vi "CheckID.vi"(8 "error in":errorcluster, 10 "CANData":T1, 11 "CAN-Frames":refnum<k21>[](array[refnum])) -> (0 "error out":errorcluster, 1 "FrameOut":T2, 2 "found？":bool)   [LabVIEW 2019, in "CAN-NI.lvlib" / "CAN-NI.lvclass"]
uses:
  CAN-NI.lvclass
  CAN-Interface/TypeDef/Def-CANData.ctl
  <resource>/objmgr/xnet.rc
  CAN-Interface/Class-Interface.lvclass
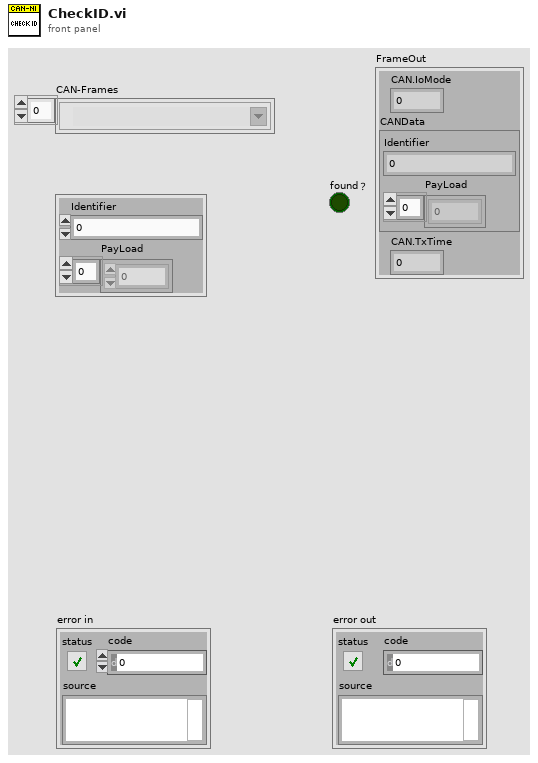
[diagram p1: front panel]
types:
  T1 = typedef "CAN-Interface.lvlib/Class-Interface.lvclass/Def-CANData.ctl" = cluster{"Identifier":u32, "PayLoad":u8[]}
  T2 = cluster{"CAN.IoMode":u32, "CANData":T1, "CAN.TxTime":dbl}
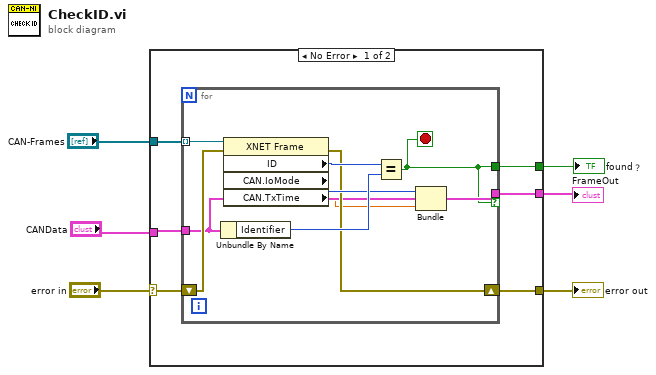
[diagram p0: block diagram]
diagram:
  n1 = case shown="No Error" "error in" {
    selector: "error in" -> [w9 w23]
    tunnel: "CAN-Frames" -> [w12 _]
    tunnel: "CANData" -> [w7 _]
    tunnel: [w11 _] -> w1
    tunnel: [w10 _] -> w5
    tunnel: [w8 w23] -> w3
    frame No Error {
      n2 = for {
        tunnel: w12 -> [w22] mode=indexing
        tunnel: [w18] -> w11 if=w15
        tunnel: [w15] -> w10
        shift-right: [w16] -> w8
        shift-left: w9 -> [w17]
        tunnel: w7 -> [w14]
        stop <- w15 stop-if-true
        n3 = Unbundle By Name(w14) -> ("Identifier"=w20:u32)
        n4 = property class="XNET Frame"(reference=w22, error in=w17) -> (error out=w16:errorcluster, "ID"=w21:u32, "CAN.IoMode"=w19:u32, "CAN.TxTime"=w13:dbl)  [unwired: 1 out]
        n5 = Equal?(x=w21, y=w20) -> (x = y?=w15:bool)
        n6 = Bundle("CAN.IoMode"=w19, "CANData"=w14, "CAN.TxTime"=w13) -> (w18:T2)  [unwired: 1 in]
      }
    }
    frame Error {
    }
  }
  "found？" <- w5
  "error out" <- w3
  "FrameOut" <- w1
